vi "Main.vi"(8 "error in":errorcluster, 11 "Device Manager in":refnum<class "Device Manager.lvclass">) -> (0 "error out":errorcluster, 3 "Device Manager out":refnum<class "Device Manager.lvclass">)   [LabVIEW 2017, in "Device Manager.lvclass"]
doc: "The <b>Queued Message Handler</b> of the Worker that owns this VI."
uses:
  Device Manager.lvclass
  C:/Program Files (x86)/National Instruments/LabVIEW 2017/vi.lib/addons/_Workers/Library/Classes/Worker/Worker.lvclass
  Device Manager.lvclass/Device Manager.ctl
  Initialization Data.ctl
  Response Cases.ctl
  Servo Motor Emulator/rqp_Set Position.ctl
  Front Panel Emulator/rqp_Update Humidity.ctl
  Front Panel Emulator/rqp_Update Temperature.ctl
  <vilib>/addons/_Workers/Library/Classes/Message Queue/Message Queue.lvclass
  Servo Motor Emulator/Servo Motor Emulator.lvclass
  Front Panel Emulator/Front Panel Emulator.lvclass
panel:
  in  "Shutdown":bool
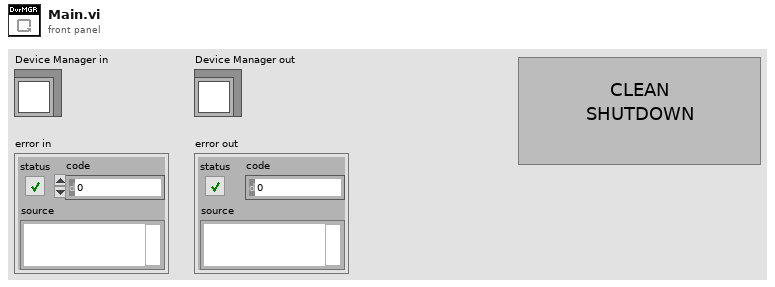
[diagram p1: front panel]
types:
  T1 = typedef "Device Manager.lvclass/Initialization Data.ctl" = cluster{"Response Cases":T2}
  T2 = typedef "Device Manager.lvclass/Response Cases.ctl" = cluster{"Placeholder - Can be deleted":string}
  T3 = typedef "Servo Motor Emulator.lvclass/rqp_Set Position.ctl" = cluster{"Position":dbl}
  T4 = typedef "Front Panel Emulator.lvclass/rqp_Update Humidity.ctl" = cluster{"Humidity":dbl}
  T5 = typedef "Front Panel Emulator.lvclass/rqp_Update Temperature.ctl" = cluster{"Temperature":dbl}
  T6 = typedef "Front Panel Emulator.lvclass/rsp_Set Position.ctl" = cluster{"Position":dbl}
  T7 = typedef "Servo Motor Emulator.lvclass/rsp_Report Humidity.ctl" = cluster{"Humidity":dbl}
  T8 = typedef "Servo Motor Emulator.lvclass/rsp_Report Temperature.ctl" = cluster{"Temperature":dbl}
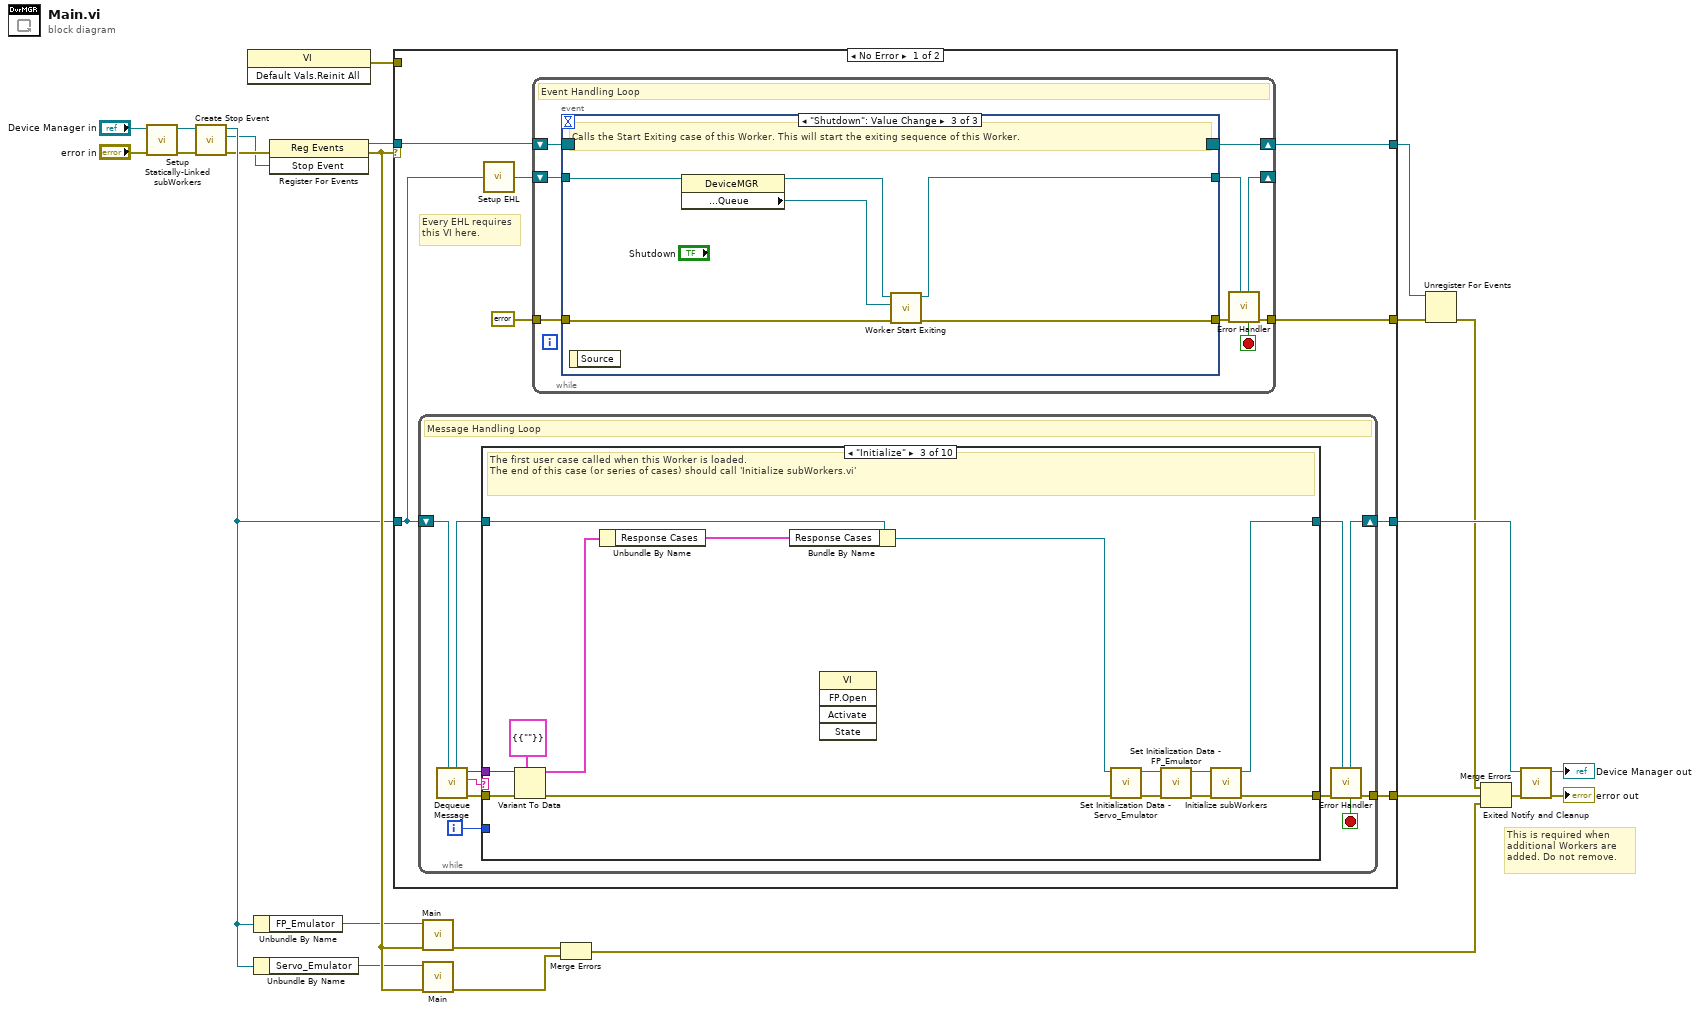
[diagram p0: block diagram]
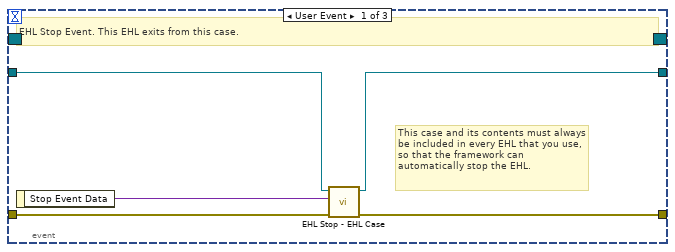
[diagram p2: hidden frame]
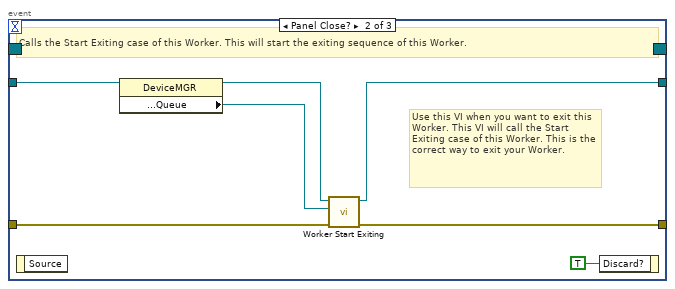
[diagram p3: hidden frame]
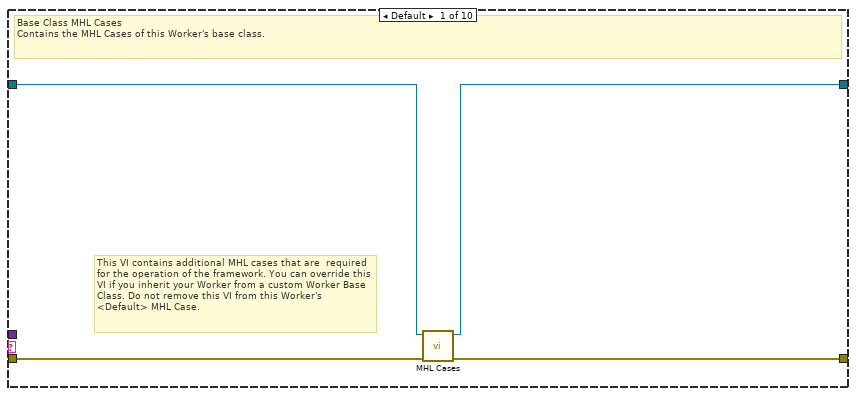
[diagram p4: hidden frame]
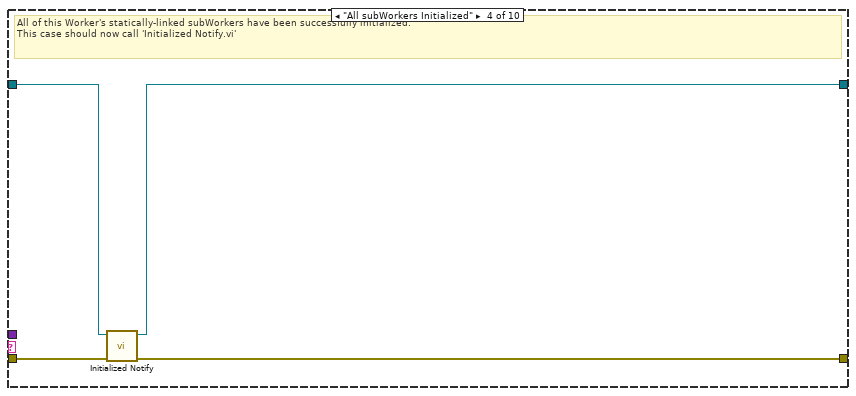
[diagram p6: hidden frame]
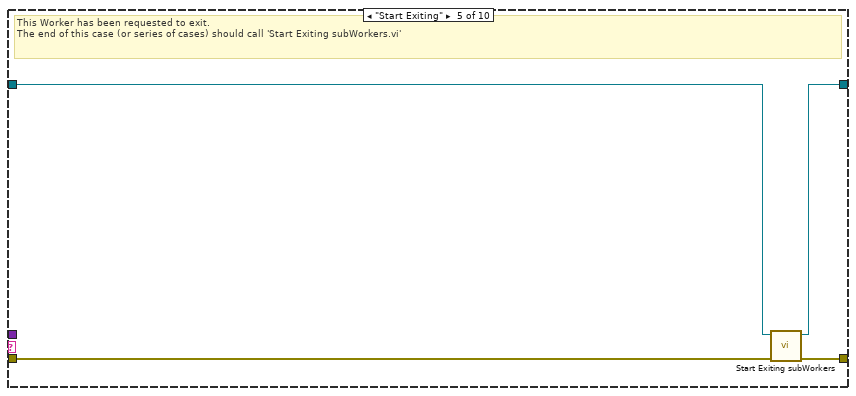
[diagram p7: hidden frame]
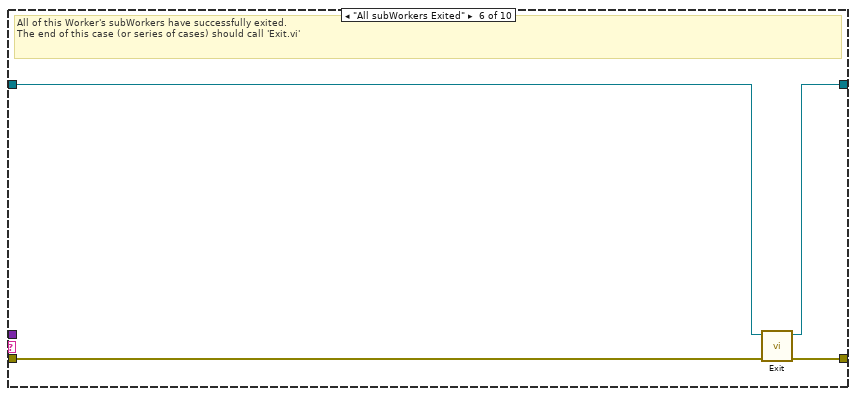
[diagram p8: hidden frame]
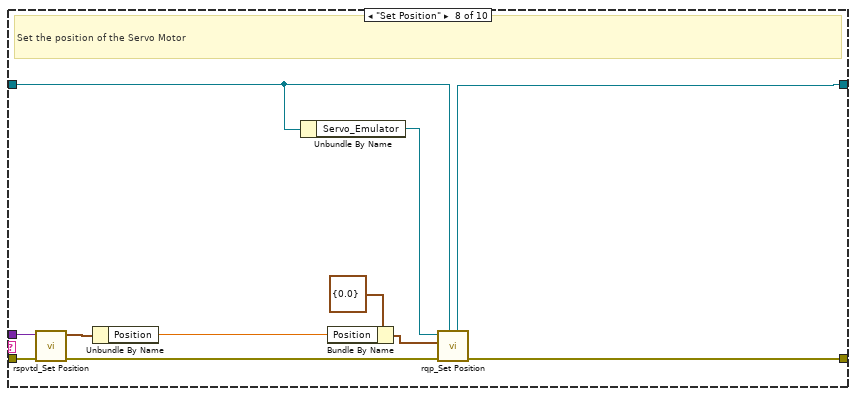
[diagram p10: hidden frame]
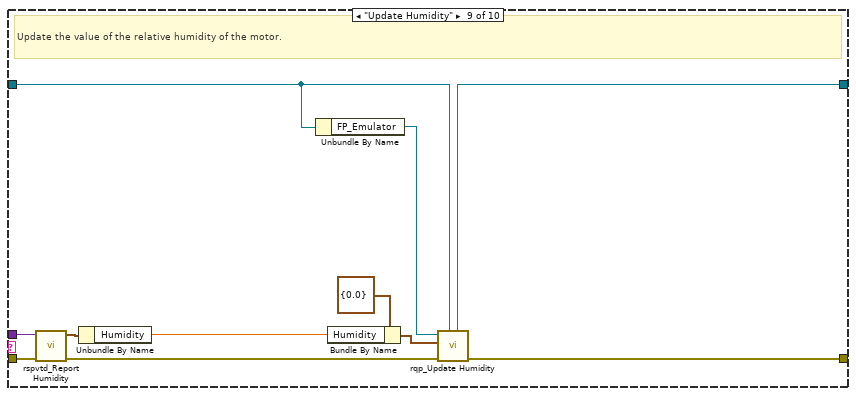
[diagram p11: hidden frame]
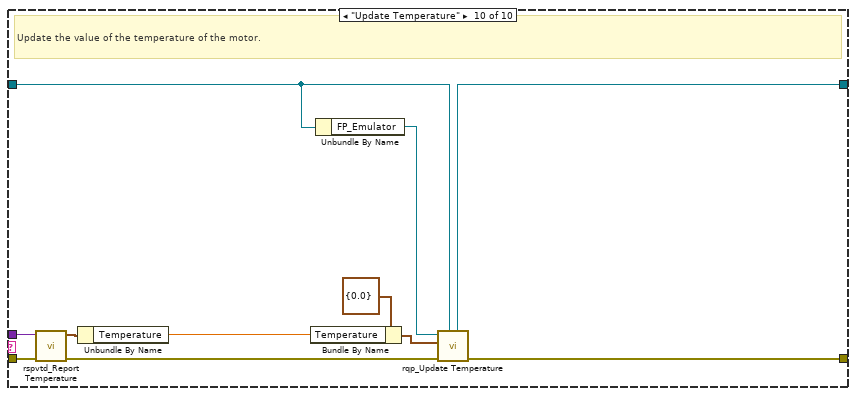
[diagram p12: hidden frame]
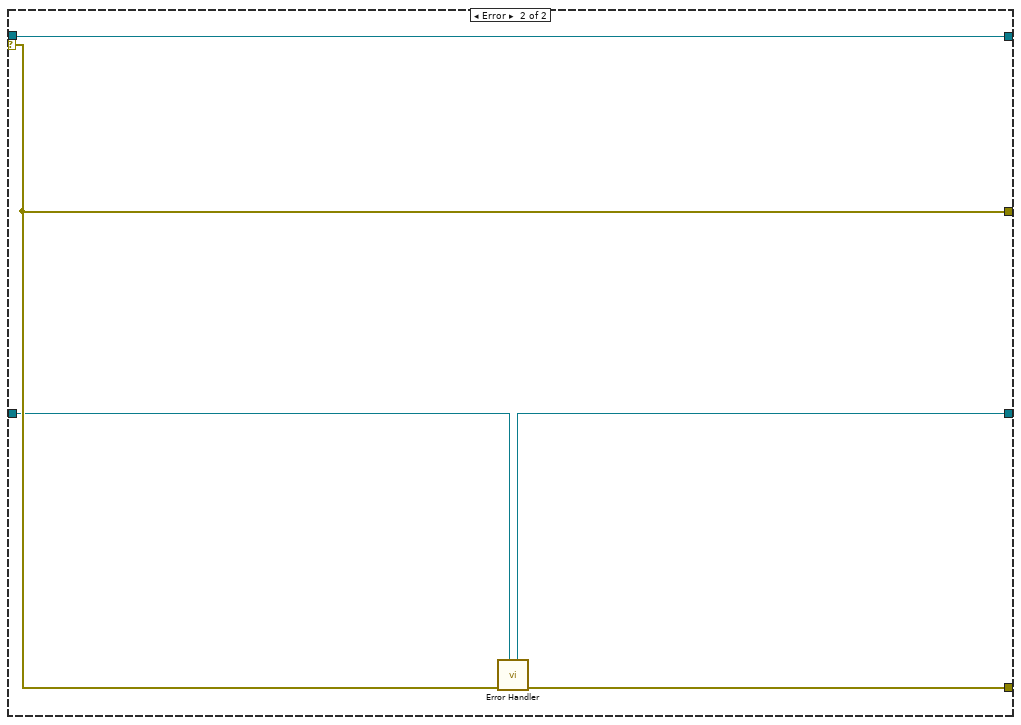
[diagram p13: hidden frame]
diagram:
  # "This is required when additional Workers are added. Do not remove."
  n1 = call "Setup Statically-Linked subWorkers.vi"("error in"="error in", "Device Manager in"="Device Manager in") -> ("error out"=w6:errorcluster, "Device Manager out"=w7:refnum<class "Device Manager.lvclass">)  [unwired: 8 in]
  n2 = call-dynamic "Create Stop Event.vi"("error in"=w6, "Worker"=w7) -> ("error out"=w9:errorcluster, "Stop Event"=w8:refnum<user-event>, "Worker out"=w15:refnum<class "Device Manager.lvclass">)  [unwired: 7 in]
  n3 = invoke class="VI" method="Default Vals.Reinit All"() -> (error out=w1:errorcluster)  [unwired: 3 in, 2 out]
  n4 = Unbundle By Name(w15) -> ("FP_Emulator"=w12:refnum<class "Front Panel Emulator.lvclass">)
  n5 = Unbundle By Name(w15) -> ("Servo_Emulator"=w10:refnum<class "Servo Motor Emulator.lvclass">)
  n6 = register-events(error in=w9, w8) -> (reference out=w5:refnum<event-registration>, error out=w17:errorcluster)  [unwired: 1 in]
  n7 = case shown="No Error" w17 {
    tunnel: w15 -> [w29 w139]
    tunnel: [w31 w140] -> w22
    tunnel: [w30 w138] -> w23
    selector: w17 -> [_ w141]
    tunnel: w5 -> [w26 w137]
    tunnel: [w25 w137] -> w4
    tunnel: [w24 w141] -> w3
    tunnel: w1 -> [_ _]
    frame No Error {
      # "Every EHL requires\nthis VI here."
      n8 = while {
        shift-right: [w67] -> w30
        shift-left: w29 -> [w69]
        tunnel: [w68] -> w31
        i -> [w59]
        stop <- w60 stop-if-true
        # "Message Handling Loop"
        n9 = call-dynamic "Dequeue Message.vi"("Worker"=w69) -> ("error out"=w66:errorcluster, "Case out"=w61:string, "Data out"=w62:variant, "Worker out"=w64:refnum<class "Device Manager.lvclass">)  [unwired: 6 in, 1 out]
        n10 = case "Worker MHL Case Structure (DO NOT CHANGE LABEL NAME)" shown="\"Initialize\"" w61 {
          tunnel: w66 -> [w73 w74 w87 w93 w94 w101 w103 w114 w125 w136]
          tunnel: [w72 w74 w89 w92 w97 w100 w103 w110 w122 w133] -> w65
          tunnel: w64 -> [w71 w75 w86 w91 w95 w99 w102 w108 w120 w131]
          tunnel: [w70 w75 w88 w90 w96 w98 w102 w109 w121 w132] -> w63
          tunnel: w62 -> [_ _ w84 _ _ _ _ w112 w123 w134]
          tunnel: w59 -> [_ _ _ _ _ _ _ _ _ _]
          frame Default {
            # "This VI contains additional MHL cases that are  required for the operation of the framework. You can override this VI if you inherit your Worker from a custom Worker Base Class. Do not remove this VI from this Worker's <Default> MHL Case."
            # "Base Class MHL Cases\nContains the MHL Cases of this Worker's base class."
            n11 = call-dynamic "MHL Cases.vi"("error in"=w73, "Worker in"=w71) -> ("error out"=w72:errorcluster, "Worker out"=w70:refnum<class "Device Manager.lvclass">)  [unwired: 8 in]
          }
          frame "------------ FRAMEWORK CASES -----------" {
            # "Start of Workers Framework Cases"
          }
          frame "Initialize" {
            # "The first user case called when this Worker is loaded.\nThe end of this case (or series of cases) should call 'Initialize subWorkers.vi'"
            n12 = Variant To Data(error in=w87, type=T1 {"Response Cases"={"Placeholder - Can be deleted"=""}} ("Cluster"), Variant=w84) -> (data=w83:T1, error out=w85:errorcluster)
            n13 = Unbundle By Name(w83) -> ("Response Cases"=w82:T2)
            n14 = Bundle By Name(cluster=w86, "Response Cases"=w82) -> (w77:refnum<class "Device Manager.lvclass">)
            n15 = invoke class="VI" method="FP.Open"() -> ()  [unwired: 5 in, 5 out]
            n16 = call "Set Initialization Data - Servo_Emulator.vi"("error in"=w85, "Device Manager in"=w77) -> ("error out"=w78:errorcluster, "Device Manager out"=w76:refnum<class "Device Manager.lvclass">)  [unwired: 8 in]
            n17 = call "Set Initialization Data - FP_Emulator.vi"("error in"=w78, "Device Manager in"=w76) -> ("error out"=w80:errorcluster, "Device Manager out"=w79:refnum<class "Device Manager.lvclass">)  [unwired: 8 in]
            n18 = call-dynamic "Initialize subWorkers.vi"("error in"=w80, "Worker"=w79) -> ("error out"=w89:errorcluster, "dup Worker out"=w88:refnum<class "Device Manager.lvclass">)  [unwired: 8 in]
          }
          frame "All subWorkers Initialized" {
            # "All of this Worker's statically-linked subWorkers have been successfully initialized.\nThis case should now call 'Initialized Notify.vi'"
            n19 = call-dynamic "Initialized Notify.vi"("error in"=w93, "Worker"=w91) -> ("error out"=w92:errorcluster, "dup Worker out"=w90:refnum<class "Device Manager.lvclass">)  [unwired: 8 in]
          }
          frame "Start Exiting" {
            # "This Worker has been requested to exit. \nThe end of this case (or series of cases) should call 'Start Exiting subWorkers.vi'"
            n20 = call-dynamic "Start Exiting subWorkers.vi"("error_in"=w94, "Worker"=w95) -> ("error out"=w97:errorcluster, "dup Worker out"=w96:refnum<class "Device Manager.lvclass">)  [unwired: 8 in]
          }
          frame "All subWorkers Exited" {
            # "All of this Worker's subWorkers have successfully exited. \nThe end of this case (or series of cases) should call 'Exit.vi'"
            n21 = call-dynamic "Exit.vi"("error_in"=w101, "Worker"=w99) -> ("error out"=w100:errorcluster, "dup Worker out"=w98:refnum<class "Device Manager.lvclass">)  [unwired: 8 in]
          }
          frame "------------- RESPONSE CASES --------------" {
            # "Start of Workers Response Cases"
          }
          frame "Set Position" {
            # "Set the position of the Servo Motor"
            n22 = call "rspvtd_Set Position.vi"("error in"=w114, "Data in"=w112) -> ("error out"=w113:errorcluster, "Data out"=w111:T6)  [unwired: 8 in]
            n23 = Unbundle By Name(w111) -> ("Position"=w104:dbl)
            n24 = Unbundle By Name(w108) -> ("Servo_Emulator"=w107:refnum<class "Servo Motor Emulator.lvclass">)
            n25 = Bundle By Name(cluster=T3 {"Position"=0.0} ("Data in"), "Position"=w104) -> (w105:T3)
            n26 = call "rqp_Set Position.vi"("Caller in"=w108, "error in"=w113, "Data in"=w105, "Servo Motor Emulator in"=w107) -> ("error out"=w110:errorcluster, "dup Caller out"=w109:refnum<class "Device Manager.lvclass">)  [unwired: 5 in, 1 out]
          }
          frame "Update Humidity" {
            # "Update the value of the relative humidity of the motor."
            n27 = call "rspvtd_Report Humidity.vi"("error in"=w125, "Data in"=w123) -> ("error out"=w124:errorcluster, "Data out"=w116:T7)  [unwired: 8 in]
            n28 = Unbundle By Name(w116) -> ("Humidity"=w115:dbl)
            n29 = Unbundle By Name(w120) -> ("FP_Emulator"=w119:refnum<class "Front Panel Emulator.lvclass">)
            n30 = Bundle By Name(cluster=T4 {"Humidity"=0.0} ("Data in"), "Humidity"=w115) -> (w117:T4)
            n31 = call "rqp_Update Humidity.vi"("Caller in"=w120, "error in"=w124, "Data in"=w117, "Front Panel Emulator in"=w119) -> ("error out"=w122:errorcluster, "dup Caller out"=w121:refnum<class "Device Manager.lvclass">)  [unwired: 5 in, 1 out]
          }
          frame "Update Temperature" {
            # "Update the value of the temperature of the motor."
            n32 = call "rspvtd_Report Temperature.vi"("error in"=w136, "Data in"=w134) -> ("error out"=w135:errorcluster, "Data out"=w127:T8)  [unwired: 8 in]
            n33 = Unbundle By Name(w127) -> ("Temperature"=w126:dbl)
            n34 = Bundle By Name(cluster=T5 {"Temperature"=0.0} ("Data in"), "Temperature"=w126) -> (w128:T5)
            n35 = Unbundle By Name(w131) -> ("FP_Emulator"=w130:refnum<class "Front Panel Emulator.lvclass">)
            n36 = call "rqp_Update Temperature.vi"("Caller in"=w131, "error in"=w135, "Data in"=w128, "Front Panel Emulator in"=w130) -> ("error out"=w133:errorcluster, "dup Caller out"=w132:refnum<class "Device Manager.lvclass">)  [unwired: 5 in, 1 out]
          }
        }
        n37 = call-dynamic "Error Handler.vi"("Worker"=w63, "error_in"=w65) -> ("error out"=w68:errorcluster, "Stop Loop"=w60:bool, "Worker out"=w67:refnum<class "Device Manager.lvclass">)  [unwired: 7 in]
      }
      n38 = call-dynamic "Setup EHL.vi"("Worker"=w29) -> ("Worker out"=w27:refnum<class "Device Manager.lvclass">)  [unwired: 14 in]
      n39 = while "Event Handling Loop" {
        shift-right: [w40] -> w25
        shift-left: w26 -> [w39]
        tunnel: [w35] -> w24
        tunnel: errorcluster {"status"=FALSE, "code"=0, "source"=""} ("error constant") -> [w37]
        shift-right: [w33] -> _
        shift-left: w27 -> [w38]
        stop <- w32 stop-if-true
        # "Event Handling Loop"
        n40 = event shown="[2] \"Shutdown\": Value Change" {
          selector: w39 -> [_ _ _]
          dyn-events: [_ _ _] -> w40
          timeout: _ -> [_ _ _]
          tunnel: [w44 w51 w53] -> w36
          tunnel: w37 -> [w45 w50 w54]
          tunnel: w38 -> [w43 w49 w57]
          tunnel: [w42 w48 w55] -> w34
          event User Event {
            # "This case and its contents must always be included in every EHL that you use, so that the framework can automatically stop the EHL."
            # "EHL Stop Event. This EHL exits from this case."
            n41 = event-data() -> ("Stop Event Data"=w41:variant)  [unwired: 1 in]
            n42 = call-dynamic "EHL Stop - EHL Case.vi"("error in"=w45, "Stop Event Data"=w41, "Worker"=w43) -> ("error out"=w44:errorcluster, "Worker out"=w42:refnum<class "Device Manager.lvclass">)  [unwired: 7 in]
          }
          event Panel Close? {
            # "Use this VI when you want to exit this Worker. This VI will call the Start Exiting case of this Worker. This is the correct way to exit your Worker."
            # "Calls the Start Exiting case of this Worker. This will start the exiting sequence of this Worker."
            n43 = event-data() -> ()  [unwired: 1 in, 1 out]
            n44 = property class="DeviceMGR"(reference=w49) -> (reference out=w47:refnum<class "Device Manager.lvclass">, "Accessors:Read:Public API:Queue"=w46:refnum<class "Message Queue.lvclass">)  [unwired: 1 in, 1 out]
            n45 = call-dynamic "Worker Start Exiting.vi"("error_in"=w50, "Message Queue"=w46, "Worker"=w47) -> ("error out"=w51:errorcluster, "dup Worker out"=w48:refnum<class "Device Manager.lvclass">)  [unwired: 7 in]
            n46 = event-data("Discard?"=TRUE) -> ()  [unwired: 1 in, 1 out]
          }
          event "Shutdown": Value Change {
            # "Calls the Start Exiting case of this Worker. This will start the exiting sequence of this Worker."
            n47 = event-data() -> ()  [unwired: 1 in, 1 out]
            n48 = property class="DeviceMGR"(reference=w57) -> (reference out=w56:refnum<class "Device Manager.lvclass">, "Accessors:Read:Public API:Queue"=w58:refnum<class "Message Queue.lvclass">)  [unwired: 1 in, 1 out]
            n49 = call-dynamic "Worker Start Exiting.vi"("error_in"=w54, "Message Queue"=w58, "Worker"=w56) -> ("error out"=w53:errorcluster, "dup Worker out"=w55:refnum<class "Device Manager.lvclass">)  [unwired: 7 in]
          }
        }
        n50 = call-dynamic "Error Handler.vi"("Worker"=w34, "error_in"=w36) -> ("error out"=w35:errorcluster, "Stop Loop"=w32:bool, "Worker out"=w33:refnum<class "Device Manager.lvclass">)  [unwired: 7 in]
      }
    }
    frame Error {
      n51 = call-dynamic "Error Handler.vi"("Worker"=w139, "error_in"=w141) -> ("error out"=w140:errorcluster, "Worker out"=w138:refnum<class "Device Manager.lvclass">)  [unwired: 7 in, 1 out]
    }
  }
  n52 = call-dynamic "Main.vi"("error in"=w17, "Front Panel Emulator in"=w12) -> ("error out"=w14:errorcluster)  [unwired: 8 in, 1 out]
  n53 = call-dynamic "Main.vi"("error in"=w17, "Servo Motor Emulator in"=w10) -> ("error out"=w11:errorcluster)  [unwired: 8 in, 1 out]
  n54 = Merge Errors(w14, w11) -> (w13:errorcluster)
  n55 = Unregister For Events(event registration refnum=w4, error in=w3) -> (error out=w2:errorcluster)
  n56 = Merge Errors(w2, w22, w13) -> (w19:errorcluster)
  n57 = call-dynamic "Exited Notify and Cleanup.vi"("error_in"=w19, "Worker"=w23) -> ("error out"=→"error out":errorcluster, "dup Worker out"=→"Device Manager out":refnum<class "Device Manager.lvclass">)  [unwired: 8 in]
